vi "MC Cycle Engine Actual State ERD.vi"(0 "GEA2 Reference In":refnum<k24>, 1 "GEA Inputs":T2 {"Destination" format="%.0x"; "Source" format="%.0x"}, 2 "Standalone?":bool, 7 "Cycle #":u8, 9 "Actual Expected State":T1, 11 "Error In":errorcluster) -> (4 "GEA2 Reference Out":refnum<k24>, 6 "Pass/Fail?":bool, 8 "Report Text":string, 15 "Error Out":errorcluster)   [LabVIEW 2016, in "2015 VA Washer.lvlib"]
doc: "This vi can be used to update the MC cycle engine state with the requested values."
uses:
  Projects/2015 VA Washer.lvlib
  C:/Automation/DLLs/PC Dot Net/GeaCommunication.dll
  Common/LabVIEW GEA2 Toolkit/LabVIEW_GEA2_Toolkit.lvlibp/type defs/Source_Destination.ctl
  type defs/MC_Cycle_Engine_Actual_State.ctl
  Common/LabVIEW GEA2 Toolkit/LabVIEW_GEA2_Toolkit.lvlibp/type defs/ERD Read Data In.ctl
  Common/LabVIEW GEA2 Toolkit/LabVIEW_GEA2_Toolkit.lvlibp/type defs/Data Type.ctl
  Common/LabVIEW GEA2 Toolkit/LabVIEW_GEA2_Toolkit.lvlibp
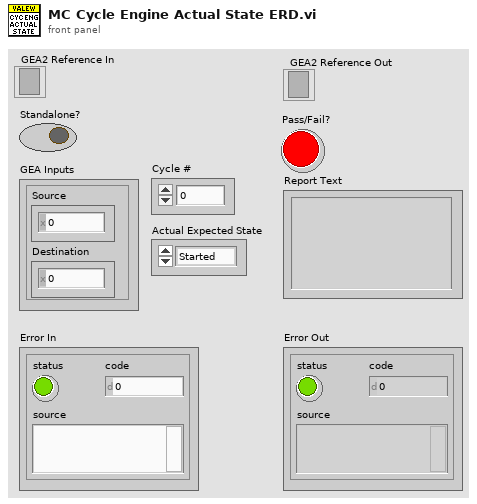
[diagram p1: front panel]
types:
  T1 = typedef "2015 VA Washer.lvlib/MC_Cycle_Engine_Actual_State.ctl" = enum16{"Started", "Stopped", "Paused", "Resumed", "Selected", "Completed"}
  T2 = typedef "LabVIEW_GEA2_Toolkit.lvlibp/Source_Destination.ctl" = cluster{"Source":u8, "Destination":u8}
  T3 = typedef "LabVIEW_GEA2_Toolkit.lvlibp/ERD Read Data In.ctl" = cluster{"ERD Number":u16, "Data Type":T4}
  T4 = typedef "LabVIEW_GEA2_Toolkit.lvlibp/Data Type.ctl" = enum16{"string", "boolean", "uint8_t", "uint16_t", "uint32_t", "uint64_t", "int8_t", "int16_t", "int32_t", "int64_t"}
  T5 = typedef "LabVIEW_GEA2_Toolkit.lvlibp/ERD Read Data Out.ctl" = cluster{"ERD Number":u16, "Data":string}
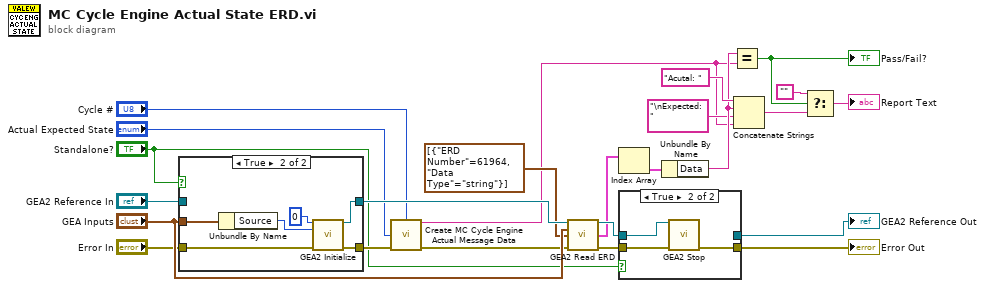
[diagram p0: block diagram]
diagram:
  n1 = case shown="True" "Standalone?" {
    tunnel: "Error In" -> [w25 w32]
    tunnel: [w25 w31] -> w21
    tunnel: "GEA2 Reference In" -> [w26 _]
    tunnel: [w26 w30] -> w19
    tunnel: "GEA Inputs" -> [_ w28]
    frame False {
    }
    frame True {
      n2 = Unbundle By Name(w28) -> ("Source"=w29:u8)
      n3 = call "GEA2 Initialize.vi"("Board Index"=0, "Source Address"=w29, "error in"=w32) -> ("GEA2 Reference Out"=w30:refnum<k24>, "error out"=w31:errorcluster)  [unwired: 10 in, 1 out]
    }
  }
  n4 = call "Create MC Cycle Engine Actual Message Data .vi"("Cycle #"="Cycle #", "MC Cycle Engine State"="Actual Expected State", "Error In"=w21) -> ("MC Cycle Engine Request Message Data"=w3:string, "Error Out"=w20:errorcluster)  [unwired: 11 in]
  n5 = call "GEA2 Read ERD.vi"("GEA2 Reference In"=w19, "GEA Inputs"="GEA Inputs", "Read ERD List"=T3[] [{"ERD Number"=61964, "Data Type"=enum."string"}], "Error In"=w20) -> ("GEA2 Reference Out"=w22:refnum<k24>, "ERD Data Out"=w10:T5[], "Error Out"=w23:errorcluster)  [unwired: 8 in, 1 out]
  n6 = Index Array(array=w10) -> (element=w9:T5)  [unwired: 1 in]
  n7 = case shown="True" "Standalone?" {
    tunnel: w23 -> [w33 w37]
    tunnel: [w33 w36] -> w17
    tunnel: w22 -> [w34 w35]
    tunnel: [w34 _] -> w16
    frame False {
    }
    frame True {
      n8 = call "GEA2 Stop.vi"("GEA2 Reference In"=w35, "Error In"=w37) -> ("Error Out"=w36:errorcluster)  [unwired: 13 in]
    }
  }
  "Error Out" <- w17
  "GEA2 Reference Out" <- w16
  n9 = Unbundle By Name(w9) -> ("Data"=w5:string)
  n10 = Equal?(x=w5, y=w3) -> (x = y?=w8:bool)
  "Pass/Fail?" <- w8
  n11 = Concatenate Strings("Acutal: " ("string"), w5, "\nExpected: " ("string"), w3) -> (w2:string)
  n12 = Select(t="", s=w8, f=w2) -> (s? t:f=→"Report Text":string)
